vi "Update Property.vi"(8 "error in (no error)":errorcluster, 9 "Value":variant, 10 "Name":string, 11 "RelationPanel in":refnum<class "RelationPanel.lvclass">) -> (0 "error out":errorcluster, 3 "RelationPanel out":refnum<class "RelationPanel.lvclass">)   [LabVIEW 2020, in "Conditum-Tools.lvlib" / "RelationPanel.lvclass"]
uses:
  RelationPanel.lvclass
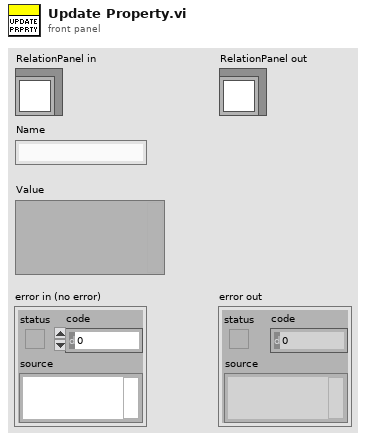
[diagram p1: front panel]
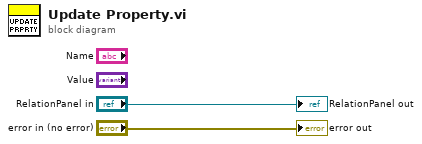
[diagram p0: block diagram]
diagram:
  "error out" <- "error in (no error)"
  "RelationPanel out" <- "RelationPanel in"
